vi "Close.vi"(8 "error in (no error)":errorcluster, 11 "File Download Controller in":refnum<class "File Download Controller.lvclass">) -> (0 "error out":errorcluster, 3 "File Download Controller out":refnum<class "File Download Controller.lvclass">)   [LabVIEW 2020, in "NI_SFTP.lvlib" / "File Download Controller.lvclass"]
uses:
  <vilib>/net/SFTP/API/Support/Download/File/File Download Controller.lvclass
  <vilib>/net/SFTP/API/Support/Download/File/File Download Controller.lvclass/File Download Controller.ctl
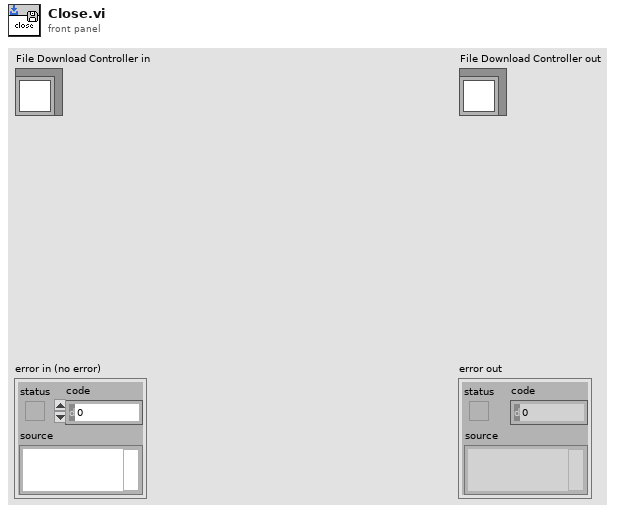
[diagram p1: front panel]
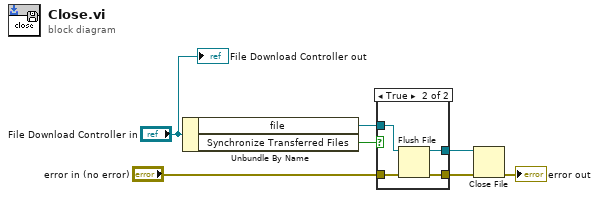
[diagram p0: block diagram]
diagram:
  n1 = Unbundle By Name("File Download Controller in") -> ("file"=w5:refnum<file>, "Synchronize Transferred Files"=w6:bool)
  n2 = case shown="True" w6 {
    tunnel: "error in (no error)" -> [w8 w13]
    tunnel: [w8 w12] -> w2
    tunnel: [w9 w11] -> w4
    tunnel: w5 -> [w9 w10]
    frame False {
    }
    frame True {
      n3 = Flush File(refnum=w10, error in=w13) -> (refnum out=w11:refnum<file>, error out=w12:errorcluster)
    }
  }
  n4 = Close File(refnum=w4, error in=w2) -> (error out=→"error out":errorcluster)  [unwired: 1 out]
  "File Download Controller out" <- "File Download Controller in"
